vi "Get MAC Address of Any Computer on Your Subnet LV2012 NI Verified plc.vi"(3 "error constant":errorcluster, 5 "IP Address":string) -> (0 "error out":errorcluster, 1 "x .and. y?":bool, 2 "MAC Address":string)   [LabVIEW 2017]
doc: "This VI uses the system exec VI to issue the command line utilities \"ping\" and \"arp\" to obtain the MAC Address of the network interface from a different computer on your network. Its functionality is limited to Windows systems.\n\nThe arp utility only works for IP addresses on the same local subnet as the computer executing the VI. Furthermore, it does not work for the IP address of the computer running the VI. This utility attempts to use the ipconfig utility for Windows NT/2000/XP to get the MAC Address of the local computer, but if the local computer's IP Address is given, it will fail when run under Windows 9x or Windows ME."
panel:
  out "after substring":string
  # "Overview: This VI uses the system exec VI to issue the command line utilities \"ping\" and \"arp\" to obtain the MAC Address of the network interface from a different computer on your network.\n\nRequirements: LabVIEW 2012 (or compatible). Hardware: network adapter.\n\nInstructions:\n1. Enter IP address in the string.\n2. Run the VI.\n3. You will receive MAC address of the adapter. Be aware of multiple network adapters."
  # "28-E9-8E-5A-D6-50"
  # "28-E9-8E-5A-D6-3B"
  # "28-E9-8E-5A-D6-59"
  # "28-E9-8E-5A-D6-5E"
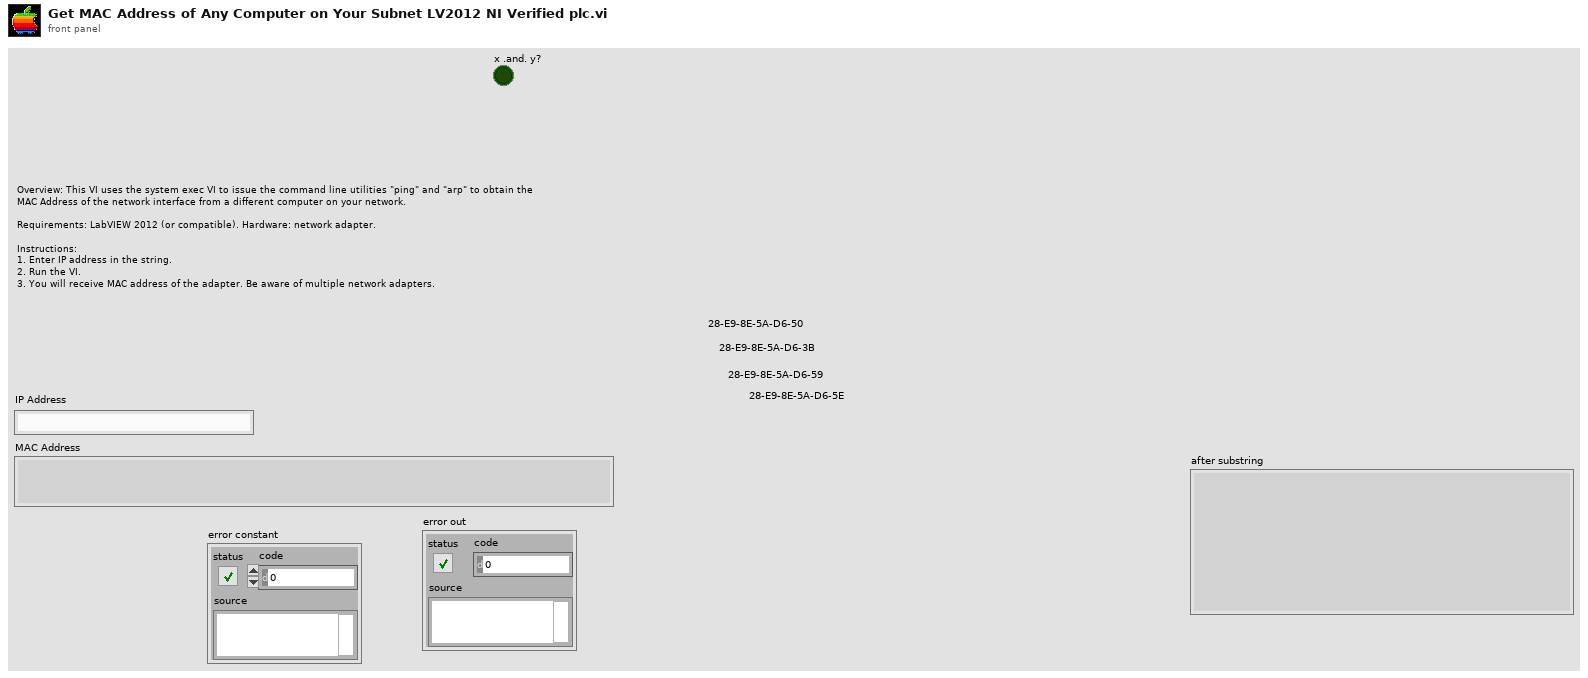
[diagram p1: front panel]
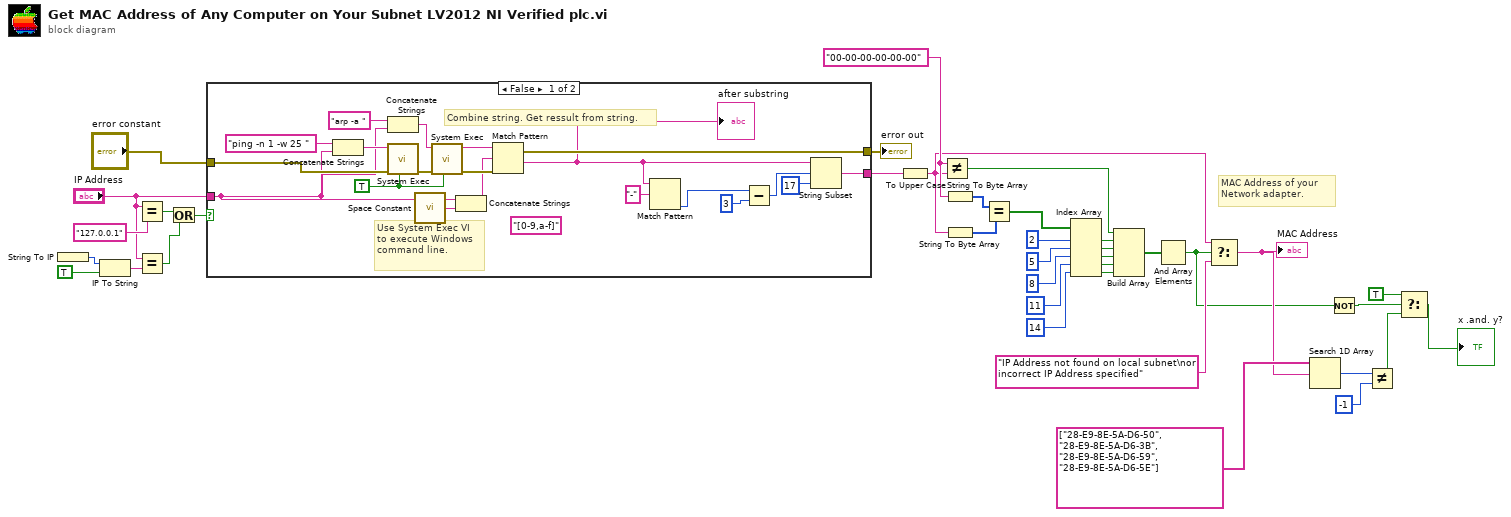
[diagram p0: block diagram]
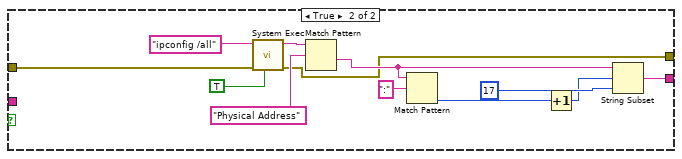
[diagram p2: hidden frame]
diagram:
  w15 = "00-00-00-00-00-00" ("regular expression")
  # "MAC Address of your\nNetwork adapter."
  n1 = String To IP() -> (0:w38:u32)  [unwired: 1 out]
  n2 = IP To String(1:TRUE ("dot notation? (F)"), 2:w38) -> (0:w35:string)
  n3 = Equal?(x="IP Address", y="127.0.0.1") -> (x = y?=w33:bool)
  n4 = Equal?(x="IP Address", y=w35) -> (x = y?=w32:bool)
  n5 = Or(x=w33, y=w32) -> (x .or. y?=w31:bool)
  n6 = case shown="False" w31 {
    tunnel: "IP Address" -> [w41 _]
    tunnel: [w48 w60] -> w13
    tunnel: "error constant" -> [w47 w59]
    tunnel: [w46 w58] -> w10
    frame False {
      w49 = TRUE ("run minimized? (F)")
      (unwired) "[0-9,a-f]" ("regular expression")
      # "Combine string. Get ressult from string."
      # "Use System Exec VI to execute Windows command line."
      n7 = Concatenate Strings("ping -n 1 -w 25 " ("command line"), w41) -> (w53:string)
      n8 = Concatenate Strings("arp -a " ("command line"), w41) -> (w54:string)
      n9 = call <vilib>:"System Exec.vi"("run minimized? (F)"=w49, "error in (no error)"=w47, "command line"=w53) -> ("error out"=w57:errorcluster)  [unwired: 3 in, 5 out]
      n10 = call <vilib>:"Space Constant.vi"() -> ("String"=w39:string)
      n11 = call <vilib>:"System Exec.vi"("run minimized? (F)"=w49, "error in (no error)"=w57, "command line"=w54) -> ("error out"=w46:errorcluster, "standard output"=w52:string)  [unwired: 3 in, 4 out]
      n12 = Concatenate Strings(w41, w39) -> (w40:string)
      n13 = Match Pattern(string=w52, regular expression=w40) -> (after substring=w42:string)  [unwired: 4 out]
      "after substring" <- w42
      n14 = Match Pattern(string=w42, regular expression="-") -> (offset past match=w44:i32)  [unwired: 4 out]
      n15 = Subtract(x=w44, y=3 ("x")) -> (x-y=w50:i32)
      n16 = String Subset(string=w42, offset (0)=w50, length (rest)=17 ("length (rest)")) -> (substring=w48:string)
    }
    frame True {
      n17 = call <vilib>:"System Exec.vi"("run minimized? (F)"=TRUE, "error in (no error)"=w59, "command line"="ipconfig /all") -> ("error out"=w58:errorcluster, "standard output"=w67:string)  [unwired: 3 in, 4 out]
      n18 = Match Pattern(string=w67, regular expression="Physical Address") -> (after substring=w64:string)  [unwired: 4 out]
      n19 = Match Pattern(string=w64, regular expression=":") -> (offset past match=w63:i32)  [unwired: 4 out]
      n20 = Increment(x=w63) -> (x+1=w61:i32)
      n21 = String Subset(string=w64, offset (0)=w61, length (rest)=17 ("length (rest)")) -> (substring=w60:string)
    }
  }
  "error out" <- w10
  n22 = To Upper Case(1:w13) -> (0:w12:string)
  n23 = Not Equal?(x=w15, y=w12) -> (x != y?=w14:bool)
  n24 = String To Byte Array(string=w15) -> (unsigned byte array=w17:u8[])
  n25 = String To Byte Array(string=w12) -> (unsigned byte array=w16:u8[])
  n26 = Equal?(x=w17, y=w16) -> (x = y?=w18:bool[])
  n27 = Index Array(array=w18, index #1=2 ("index"), index #2=5 ("index"), index #3=8 ("index"), index #4=11 ("index"), index #5=14 ("index")) -> (element #1=w28:bool, element #2=w27:bool, element #3=w26:bool, element #4=w25:bool, element #5=w24:bool)
  n28 = Build Array(w14, w28, w27, w26, w25, w24) -> (w29:bool[])
  n29 = And Array Elements(Boolean array=w29) -> (logical AND=w5:bool)
  n30 = Select(t=w12, s=w5, f="IP Address not found on local subnet\nor incorrect IP Address specified") -> (s? t:f=w8:string)
  "MAC Address" <- w8
  n31 = Search 1D Array(1D array=string[] ["28-E9-8E-5A-D6-50", "28-E9-8E-5A-D6-3B", "28-E9-8E-5A-D6-59", "28-E9-8E-5A-D6-5E"], element=w8) -> (index of element=w7:i32)  [unwired: 1 in]
  n32 = Not(x=w5) -> (.not. x?=w4:bool)
  n33 = Not Equal?(x=w7, y=-1) -> (x != y?=w3:bool)
  n34 = Select(t=TRUE, s=w4, f=w3) -> (s? t:f=→"x .and. y?":bool)
